vi "Write Sleep TS.vi"(8 "error in (no error)":errorcluster, 10 "Sleep":i64, 11 "CIFCorePlugin in":refnum<class "CIFCorePlugin.lvclass">) -> (0 "error out":errorcluster, 3 "CIFCorePlugin out":refnum<class "CIFCorePlugin.lvclass">)   [LabVIEW 2021, in "CIFCorePlugin.lvclass"]
doc: "Update the timestamp. Time is U64, absolute time in nS in the appropriate clockID configured for the plugin. If a 0 is wired it will automatically get the current time."
uses:
  CIFCorePlugin.lvclass
  CIFCorePlugin.lvclass/CIFCorePlugin.ctl
  <vilib>/CIF Foundation/CIF Utilities/Time/System Time/LabVIEW Time to TAI Time.vi
  <vilib>/CIF Foundation/CIF Utilities/Time/Time_CIF_U.lvlib
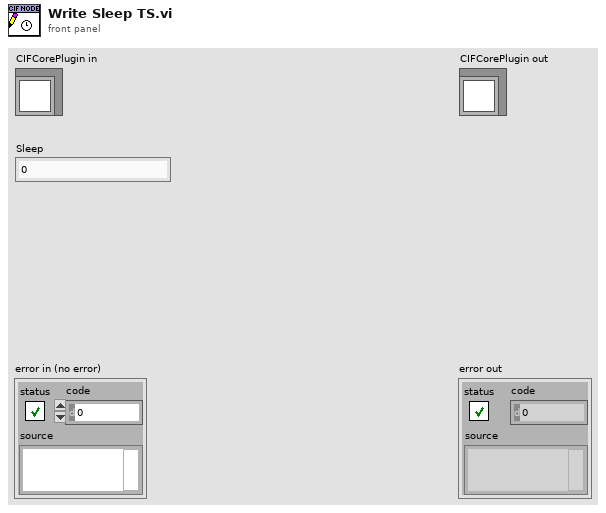
[diagram p1: front panel]
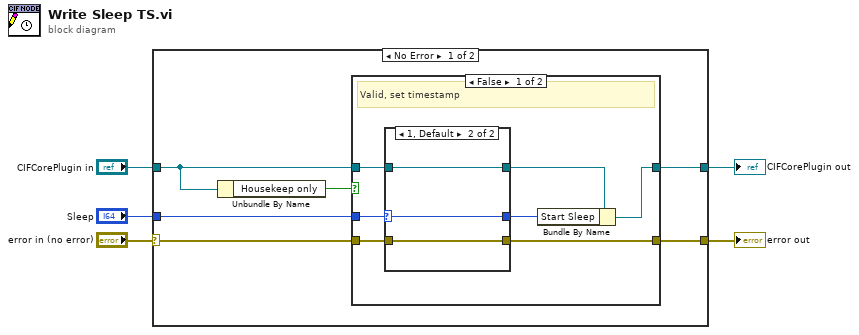
[diagram p0: block diagram]
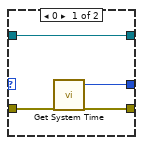
[diagram p2: hidden frame]
diagram:
  n1 = case shown="No Error" "error in (no error)" {
    selector: "error in (no error)" -> [w9 w27]
    tunnel: [w8 w27] -> w4
    tunnel: [w11 w28] -> w2
    tunnel: "CIFCorePlugin in" -> [w7 w28]
    tunnel: "Sleep" -> [w10 _]
    frame No Error {
      n2 = Unbundle By Name(w7) -> ("Housekeep only"=w6:bool)
      n3 = case shown="False" w6 {
        tunnel: [w18 w26] -> w11
        tunnel: w10 -> [w17 _]
        tunnel: w9 -> [w16 w25]
        tunnel: [w13 w25] -> w8
        tunnel: w7 -> [w12 w26]
        frame False {
          # "Valid, set timestamp"
          n4 = case shown="1, Default" w17 {
            selector: w17 -> [_ w23]
            tunnel: w16 -> [w19 w22]
            tunnel: w12 -> [w21 w24]
            tunnel: [w21 w24] -> w15
            tunnel: [w20 w23] -> w14
            tunnel: [w19 w22] -> w13
            frame 0 {
              n5 = call <vilib>:"Get System Time.vi"() -> ("Time (ns)"=w20:i64)  [unwired: 5 in]
            }
            frame 1, Default {
            }
          }
          n6 = Bundle By Name(cluster=w15, "Start Sleep"=w14) -> (w18:refnum<class "CIFCorePlugin.lvclass">)
        }
        frame True {
          # "Last cycle was housekeeping only, don't set timestamp for benchmark"
        }
      }
    }
    frame Error {
    }
  }
  "error out" <- w4
  "CIFCorePlugin out" <- w2
